vi "test_Packet_SimpleTrackedTarget.vi"(8 "error in (no error)":errorcluster) -> (0 "error out":errorcluster, 3 "Test Passed":bool)   [LabVIEW 2020]
uses:
  PhotonVisionLib/PhotonVisionLib.lvlib
  <vilib>/Rock Robotics/WPI/ThirdParty/JAS_Junk/TrajLib/Trajectory_Library.lvlib
  PhotonVisionLib/TypeDef/TargetCornerType.ctl
  <vilib>/Rock Robotics/WPI/ThirdParty/JAS_Junk/TrajLib/TypeDef/TRANSLATION2D.ctl
  <vilib>/Rock Robotics/WPI/ThirdParty/JAS_Junk/TrajLib/TypeDef/ROTATION2D.ctl
  <vilib>/Rock Robotics/WPI/ThirdParty/JAS_Junk/TrajLib/TypeDef/TRANSFORM2D.ctl
  PhotonVisionLib/TypeDef/PhotonTrackedTargetType.ctl
panel:
  out "TrackedTarget 2":T1={"Yaw"=0.0, "Pitch"=0.0, "Area"=0.0, "Skew"=0.0, "TargetCorners"=[], "CameraToTarget"={"TRANSLATION"={"X"=0.0, "Y"=0.0}, "ROTATION"={"VALUE"=0.0, "COS"=1.0, "SIN"=0.0}, "xF"=FALSE}, "FiducialId"=0} {"CameraToTarget"."ROTATION"."SIN" format="%13.4f"; "CameraToTarget"."ROTATION"."COS" format="%13.4f"; "CameraToTarget"."ROTATION"."VALUE" format="%13.4f"; "CameraToTarget"."TRANSLATION"."Y" format="%14.3f"; "CameraToTarget"."TRANSLATION"."X" format="%14.3f"}
  out "TrackedTarget":T1={"Yaw"=0.0, "Pitch"=0.0, "Area"=0.0, "Skew"=0.0, "TargetCorners"=[], "CameraToTarget"={"TRANSLATION"={"X"=0.0, "Y"=0.0}, "ROTATION"={"VALUE"=0.0, "COS"=1.0, "SIN"=0.0}, "xF"=FALSE}, "FiducialId"=0} {"CameraToTarget"."ROTATION"."SIN" format="%13.4f"; "CameraToTarget"."ROTATION"."COS" format="%13.4f"; "CameraToTarget"."ROTATION"."VALUE" format="%13.4f"; "CameraToTarget"."TRANSLATION"."Y" format="%14.3f"; "CameraToTarget"."TRANSLATION"."X" format="%14.3f"}
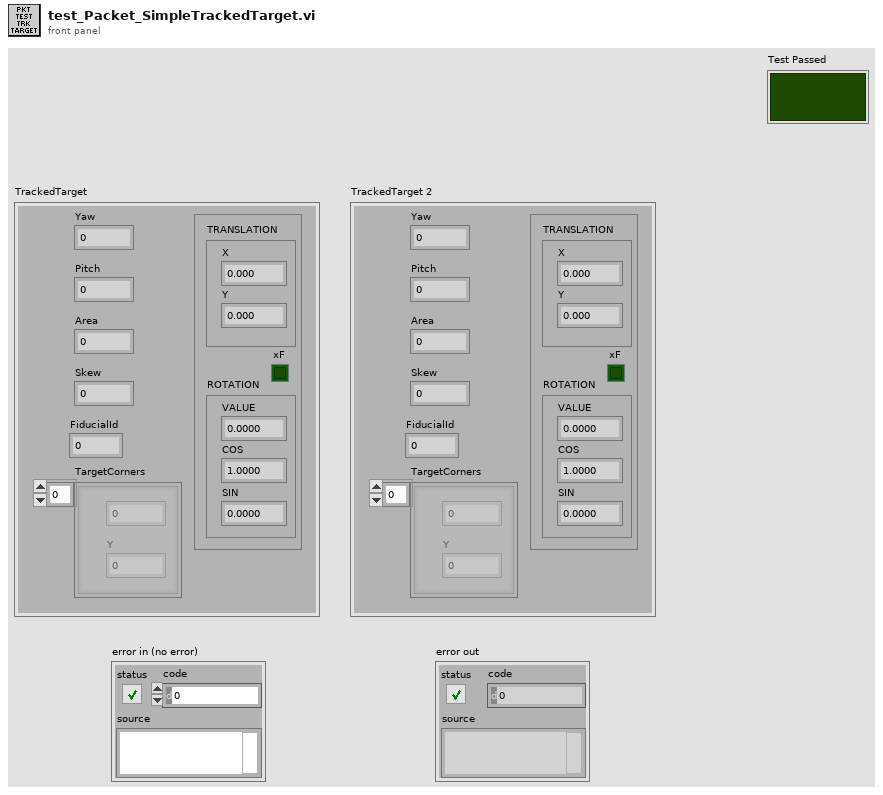
[diagram p1: front panel]
types:
  T1 = typedef "PhotonVisionLib.lvlib/PhotonTrackedTargetType.ctl" = cluster{"Yaw":dbl, "Pitch":dbl, "Area":dbl, "Skew":dbl, "TargetCorners":T2[], "CameraToTarget":T3, "FiducialId":i32}
  T2 = typedef "PhotonVisionLib.lvlib/TargetCornerType.ctl" = cluster{"X":dbl, "Y":dbl}
  T3 = typedef "Trajectory_Library.lvlib/TRANSFORM2D.ctl" = cluster{"TRANSLATION":T4, "ROTATION":T5, "xF":bool}
  T4 = typedef "Trajectory_Library.lvlib/TRANSLATION2D.ctl" = cluster{"X":dbl, "Y":dbl}
  T5 = typedef "Trajectory_Library.lvlib/ROTATION2D.ctl" = cluster{"VALUE":dbl, "COS":dbl, "SIN":dbl}
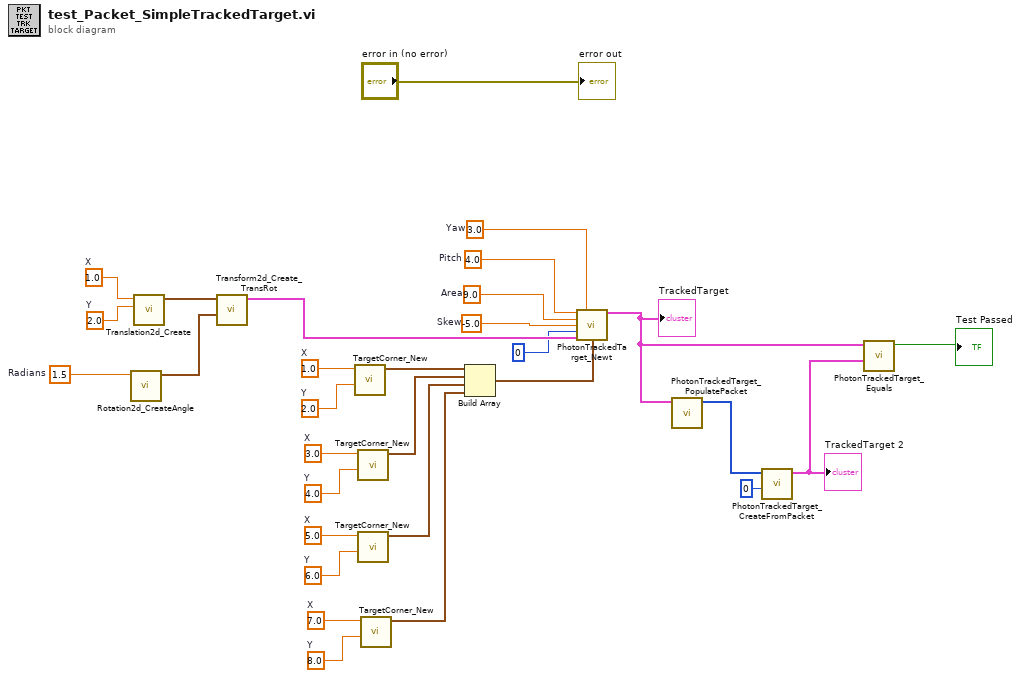
[diagram p0: block diagram]
diagram:
  w8 = 1.0  # X
  w9 = 2.0  # Y
  w11 = 1.5  # Radians
  w13 = 4.0  # Pitch
  w14 = 9.0  # Area
  w15 = -5.0  # Skew
  w16 = 3.0  # Yaw
  w22 = 7.0  # X
  w23 = 8.0  # Y
  w24 = 5.0  # X
  w25 = 6.0  # Y
  w26 = 3.0  # X
  w27 = 4.0  # Y
  w28 = 1.0  # X
  w29 = 2.0  # Y
  n1 = call <vilib>:"Rotation2d_CreateAngle.vi"("Angle"=w11) -> ("ROTATION"=w10:T5)  [unwired: 10 in]
  n2 = call <vilib>:"Translation2d_Create.vi"("Y"=w9, "X"=w8) -> ("TRANSLATION"=w12:T4)  [unwired: 9 in]
  n3 = call <vilib>:"Transform2d_Create_TransRot.vi"("ROTATION"=w10, "TRANSLATION"=w12) -> ("TRANSFORM"=w7:T3)  [unwired: 9 in]
  n4 = call "TargetCorner_New.vi"("Y"=w29, "X"=w28) -> ("TargetCorner"=w21:T2)  [unwired: 9 in]
  n5 = call "TargetCorner_New.vi"("Y"=w27, "X"=w26) -> ("TargetCorner"=w19:T2)  [unwired: 9 in]
  n6 = call "TargetCorner_New.vi"("Y"=w25, "X"=w24) -> ("TargetCorner"=w18:T2)  [unwired: 9 in]
  n7 = call "TargetCorner_New.vi"("Y"=w23, "X"=w22) -> ("TargetCorner"=w17:T2)  [unwired: 9 in]
  n8 = Build Array(w21, w19, w18, w17) -> (w20:T2[])
  n9 = call "PhotonTrackedTarget_Newt.vi"("Pitch"=w13, "Yaw"=w16, "Area"=w14, "Skew"=w15, "FiducalId"=0, "CameraToTarget"=w7, "TargetCorners"=w20) -> ("TrackedTarget"=w4:T1)  [unwired: 8 in]
  "TrackedTarget" <- w4
  n10 = call "PhotonTrackedTarget_PopulatePacket.vi"("TrackedTarget"=w4) -> ("RawData Out"=w6:u8[])  [unwired: 10 in]
  n11 = call "PhotonTrackedTarget_CreateFromPacket.vi"("StartByte"=0, "RawData"=w6) -> ("TrackedTarget"=w3:T1)  [unwired: 8 in, 1 out]
  "TrackedTarget 2" <- w3
  n12 = call "PhotonTrackedTarget_Equals.vi"("Other TrackedTarget"=w3, "TrackedTarget"=w4) -> ("Equals"=→"Test Passed":bool)  [unwired: 9 in]
  "error out" <- "error in (no error)"
